vi "Read (Math).vi"(8 "error in (no error)":errorcluster, 10 "Reset After Read (False)":bool, 11 "VISA resource name":refnum<visa-resource-name>) -> (0 "error out":errorcluster, 1 "Count":dbl, 2 "Average":dbl, 3 "VISA resource name out":refnum<visa-resource-name>, 4 "Standard Deviation":dbl, 5 "Minimum":dbl, 6 "Peak-to-Peak":dbl, 7 "Maximum":dbl)   [LabVIEW 2011, in "Agilent 34401.lvlib"]
doc: "Read (Math) returns the minimum, maximum, average, count, peak-to-peak, and standard deviation values from multiple measurements. This VI requires that Min/Max is set in Configure Math and should be called after multiple measurements have been taken.\n\n<B>Note:</B>\n\nThe Agilent 34401 does not support peak-to-peak and standard deviation values."
uses:
  Agilent 34401.lvlib
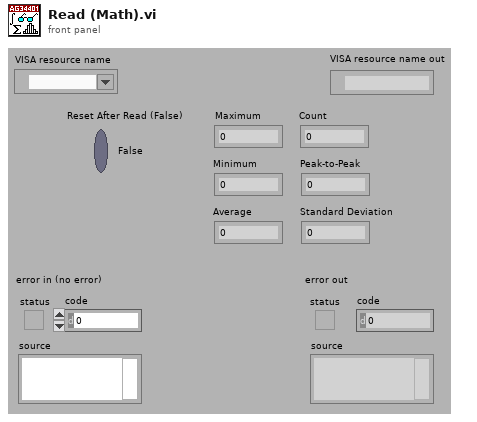
[diagram p1: front panel]
types:
  T1 = typedef "Agilent 34401.lvlib/Extended User Data.ctl" = cluster{"Trigger Source":u16, "Math Storage":u16, "Agilent Model":i32}
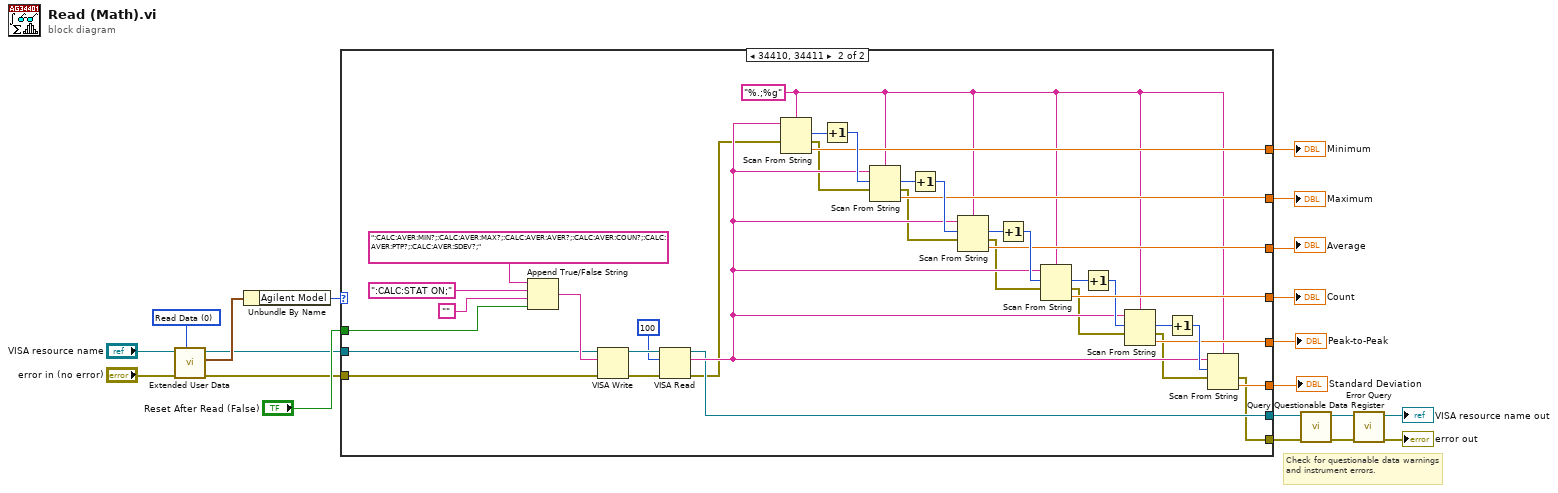
[diagram p0: block diagram]
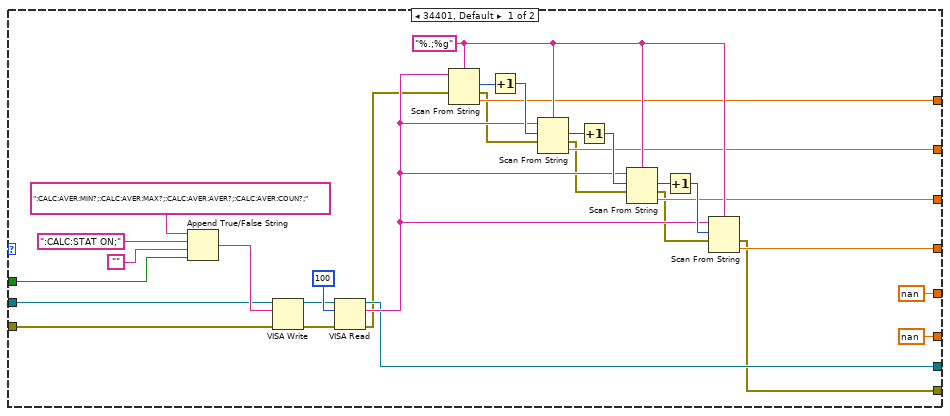
[diagram p2: hidden frame]
diagram:
  w10 = u16 0 items=["Read Data", "Write Data", "Dispose of Data"] ("Action")
  # "Check for questionable data warnings and instrument errors."
  n1 = call "Extended User Data.vi"("Action"=w10, "Error In (no error)"="error in (no error)", "VISA resource name in"="VISA resource name") -> ("Error Out"=w8:errorcluster, "User Data Out"=w11:T1, "VISA resource name out"=w7:refnum<visa-resource-name>)  [unwired: 6 in]
  n2 = Unbundle By Name(w11) -> ("Agilent Model"=w5:i32)
  n3 = case shown="34410, 34411" w5 {
    tunnel: w7 -> [w42 w79]
    tunnel: w8 -> [w43 w78]
    tunnel: "Reset After Read (False)" -> [w41 w77]
    tunnel: [w29 w70] -> w17
    tunnel: [w30 w69] -> w16
    tunnel: [w31 w68] -> w15
    tunnel: [w32 w67] -> w14
    tunnel: [nan w62] -> w13
    tunnel: [nan w61] -> w12
    tunnel: [w26 w58] -> w2
    tunnel: [w21 w51] -> w1
    frame 34401, Default {
      w34 = "%.;%g" ("format string")
      n4 = Append True/False String(1:w41, 2:"" ("Empty String Constant"), 3:":CALC:STAT ON;", 4:":CALC:AVER:MIN?;:CALC:AVER:MAX?;:CALC:AVER:AVER?;:CALC:AVER:COUN?;") -> (0:w47:string)
      n5 = VISA Write(VISA resource name=w42, write buffer=w47, error in (no error)=w43) -> (VISA resource name out=w44:refnum<visa-resource-name>, error out=w45:errorcluster)  [unwired: 1 out]
      n6 = VISA Read(VISA resource name=w44, byte count=u32 100, error in (no error)=w45) -> (VISA resource name out=w26:refnum<visa-resource-name>, read buffer=w33:string, error out=w25:errorcluster)  [unwired: 1 out]
      n7 = Scan From String(format string=w34, input string=w33, error in=w25) -> (offset past scan=w35:u32, error out=w24:errorcluster, output 1=w29:dbl)  [unwired: 2 in, 1 out]
      n8 = Increment(x=w35) -> (x+1=w36:u32)
      n9 = Scan From String(format string=w34, input string=w33, initial scan location=w36, error in=w24) -> (offset past scan=w37:u32, error out=w23:errorcluster, output 1=w30:dbl)  [unwired: 1 in, 1 out]
      n10 = Increment(x=w37) -> (x+1=w38:u32)
      n11 = Scan From String(format string=w34, input string=w33, initial scan location=w38, error in=w23) -> (offset past scan=w39:u32, error out=w22:errorcluster, output 1=w31:dbl)  [unwired: 1 in, 1 out]
      n12 = Increment(x=w39) -> (x+1=w40:u32)
      n13 = Scan From String(format string=w34, input string=w33, initial scan location=w40, error in=w22) -> (error out=w21:errorcluster, output 1=w32:dbl)  [unwired: 1 in, 2 out]
    }
    frame 34410, 34411 {
      w60 = "%.;%g" ("format string")
      n14 = Append True/False String(1:w77, 2:"" ("Empty String Constant"), 3:":CALC:STAT ON;", 4:":CALC:AVER:MIN?;:CALC:AVER:MAX?;:CALC:AVER:AVER?;:CALC:AVER:COUN?;:CALC:AVER:PTP?;:CALC:AVER:SDEV?;") -> (0:w83:string)
      n15 = VISA Write(VISA resource name=w79, write buffer=w83, error in (no error)=w78) -> (VISA resource name out=w86:refnum<visa-resource-name>, error out=w85:errorcluster)  [unwired: 1 out]
      n16 = VISA Read(VISA resource name=w86, byte count=u32 100, error in (no error)=w85) -> (VISA resource name out=w58:refnum<visa-resource-name>, read buffer=w59:string, error out=w57:errorcluster)  [unwired: 1 out]
      n17 = Scan From String(format string=w60, input string=w59, error in=w57) -> (offset past scan=w71:u32, error out=w56:errorcluster, output 1=w70:dbl)  [unwired: 2 in, 1 out]
      n18 = Increment(x=w71) -> (x+1=w72:u32)
      n19 = Scan From String(format string=w60, input string=w59, initial scan location=w72, error in=w56) -> (offset past scan=w73:u32, error out=w55:errorcluster, output 1=w69:dbl)  [unwired: 1 in, 1 out]
      n20 = Increment(x=w73) -> (x+1=w74:u32)
      n21 = Scan From String(format string=w60, input string=w59, initial scan location=w74, error in=w55) -> (offset past scan=w75:u32, error out=w54:errorcluster, output 1=w68:dbl)  [unwired: 1 in, 1 out]
      n22 = Increment(x=w75) -> (x+1=w76:u32)
      n23 = Scan From String(format string=w60, input string=w59, initial scan location=w76, error in=w54) -> (offset past scan=w66:u32, error out=w53:errorcluster, output 1=w67:dbl)  [unwired: 1 in, 1 out]
      n24 = Increment(x=w66) -> (x+1=w65:u32)
      n25 = Scan From String(format string=w60, input string=w59, initial scan location=w65, error in=w53) -> (offset past scan=w64:u32, error out=w52:errorcluster, output 1=w62:dbl)  [unwired: 1 in, 1 out]
      n26 = Increment(x=w64) -> (x+1=w63:u32)
      n27 = Scan From String(format string=w60, input string=w59, initial scan location=w63, error in=w52) -> (error out=w51:errorcluster, output 1=w61:dbl)  [unwired: 1 in, 2 out]
    }
  }
  "Minimum" <- w17
  "Maximum" <- w16
  "Average" <- w15
  "Count" <- w14
  "Peak-to-Peak" <- w13
  "Standard Deviation" <- w12
  n28 = call "Query Questionable Data Register.vi"("error in (no error)"=w1, "VISA resource name"=w2) -> ("error out"=w4:errorcluster, "VISA resource name out"=w3:refnum<visa-resource-name>)  [unwired: 7 in, 1 out]
  n29 = call "Error Query.vi"("error in (no error)"=w4, "VISA resource name"=w3) -> ("error out"=→"error out":errorcluster, "VISA resource name out"=→"VISA resource name out":refnum<visa-resource-name>)  [unwired: 6 in, 2 out]
